vi "Read Results in Filename.vi"(8 "error in (no error)":errorcluster, 11 "POLARIS TA Focus Display in":refnum<class "POLARIS TA Focus Display.lvclass">) -> (0 "error out":errorcluster, 2 "Results in Filename":bool, 3 "POLARIS TA Focus Display out":refnum<class "POLARIS TA Focus Display.lvclass">)   [LabVIEW 2014, in "POLARIS TA Focus Display.lvlib" / "POLARIS TA Focus Display.lvclass"]
uses:
  POLARIS TA Focus Display.lvclass
  POLARIS TA Focus Display.lvclass/POLARIS TA Focus Display.ctl
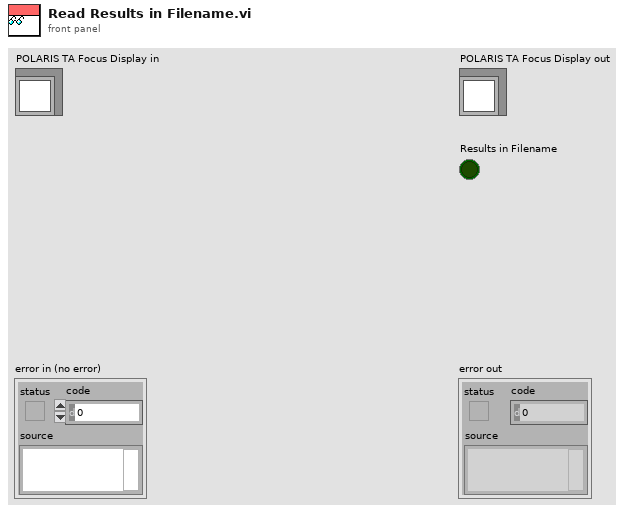
[diagram p1: front panel]
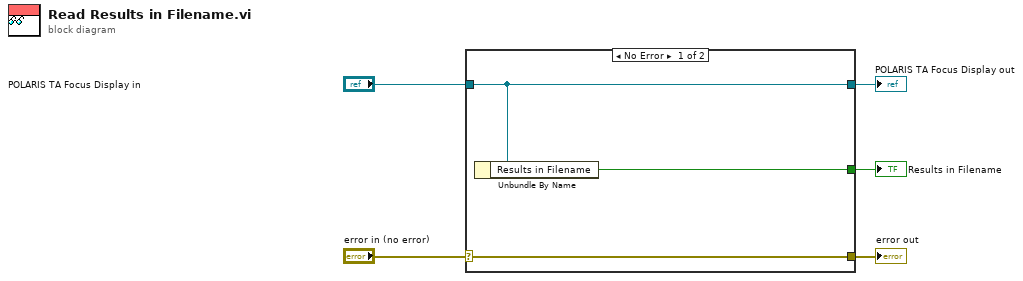
[diagram p0: block diagram]
diagram:
  n1 = case shown="No Error" "error in (no error)" {
    selector: "error in (no error)" -> [w8 w9]
    tunnel: [w8 w9] -> w4
    tunnel: [w7 w10] -> w2
    tunnel: "POLARIS TA Focus Display in" -> [w7 w10]
    tunnel: [w6 _] -> w1
    frame No Error {
      n2 = Unbundle By Name(w7) -> ("Results in Filename"=w6:bool)
    }
    frame Error {
    }
  }
  "error out" <- w4
  "POLARIS TA Focus Display out" <- w2
  "Results in Filename" <- w1
